vi "TestKinematics.vi"() -> ()   [LabVIEW 2016]
uses:
  <vilib>/robotics/Steering/Wheel/Wheel State.ctl
  MotorControl/Configurations.ctl
  <vilib>/robotics/Steering/Wheel/Wheel Parameters.ctl
  <vilib>/robotics/Steering/Wheel/Rotation Direction.ctl
  <vilib>/robotics/Steering/Differential Steering Frame/NI_Robotics_Differential Steering Frame.lvclass
  C:/Program Files (x86)/National Instruments/LabVIEW 2016/vi.lib/robotics/Steering/Steering Frame/NI_Robotics_Steering Frame.lvclass
  <vilib>/robotics/Steering/Steering Frame/Apply Steering Frame Velocity to Wheels.vi
  <vilib>/robotics/Steering/Steering Frame/NI_Robotics_Steering Frame.lvclass
  C:/Program Files (x86)/National Instruments/LabVIEW 2016/vi.lib/robotics/Steering/Special Steering Frame/NI_Robotics_Special Steering Frame.lvclass
  <vilib>/robotics/Steering/Wheel/NI_Robotics_Wheel.lvclass
panel:
  in  "Robot Configuration":T1={"wheel parameters"={"wheel radius"=0.1, "gear ratio"=1.0, "forward rotation direction"=0}, "wheel separation"=0.4, "Encoder Pulse Per Rev"=1920.0} {"wheel parameters"."forward rotation direction" items=["Clockwise", "Counterclockwise"]}
  out "calculated wheel states":T4[](array[typedef])
  in  "stop":bool
  in  "steering frame velocity":dbl[](array[numeric])=[0.0, 0.0, 0.0]
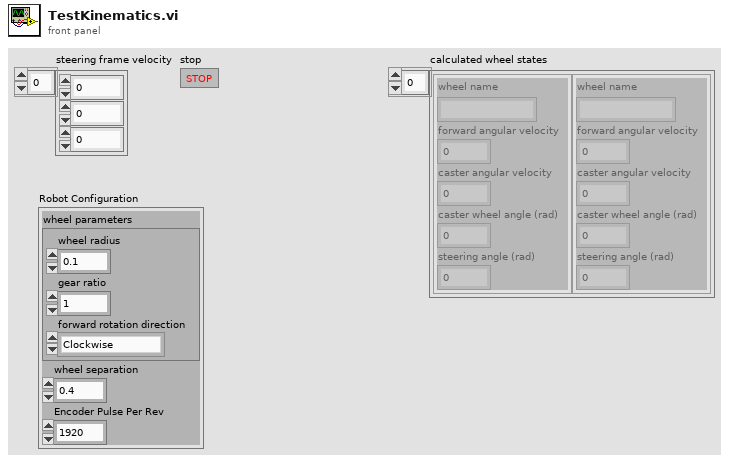
[diagram p1: front panel]
types:
  T1 = typedef "Configurations.ctl" = cluster{"wheel parameters":T2, "wheel separation":dbl, "Encoder Pulse Per Rev":dbl}
  T2 = typedef "NI_Robotics_Wheel.lvclass/Wheel Parameters.ctl" = cluster{"wheel radius":dbl, "gear ratio":dbl, "forward rotation direction":T3}
  T3 = typedef "NI_Robotics_Wheel.lvclass/Rotation Direction.ctl" = u16
  T4 = typedef "NI_Robotics_Wheel.lvclass/Wheel State.ctl" = cluster{"wheel name":string, "forward angular velocity":dbl, "caster angular velocity":dbl, "caster wheel angle (rad)":dbl, "steering angle (rad)":dbl}
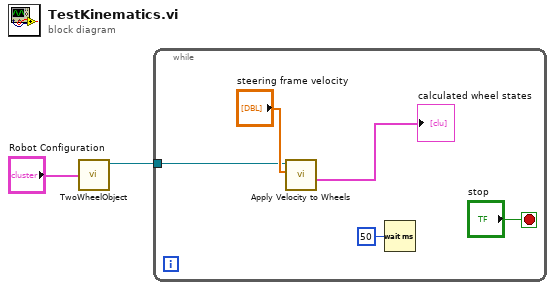
[diagram p0: block diagram]
diagram:
  n1 = call "TwoWheelObject.vi"("Robot Configuration"="Robot Configuration") -> ("differential steering frame out"=w2:refnum<class "NI_Robotics_Differential Steering Frame.lvclass">)  [unwired: 9 in, 1 out]
  n2 = while {
    tunnel: w2 -> [w3]
    stop <- "stop" stop-if-true
    n3 = call-poly <vilib>:"Apply Velocity to Wheels.vi"("steering frame velocity"="steering frame velocity", "steering frame in"=w3) -> ("calculated wheel states"=→"calculated wheel states":T4[])  [unwired: 6 in, 3 out]
    n4 = Wait (ms)(milliseconds to wait=u32 50) -> ()  [unwired: 1 out]
  }
